vi "Router - PXImc Close.vi"(8 "error in (no error)":errorcluster, 11 "Router Data In":T1) -> (0 "error out":errorcluster)   [LabVIEW 2016, in "PXImc Router.lvlib"]
uses:
  PXImc Router.lvlib
  Controls/Router - Configuration.ctl
  Controls/Router/Node Block R-W Properties.ctl
  Controls/Router/Block Properties.ctl
  Controls/Router/Router - PXImc Properties.ctl
  Controls/Router/Router - PXImc Card Properties.ctl
  <vilib>/pximc/nipximc.lvlib
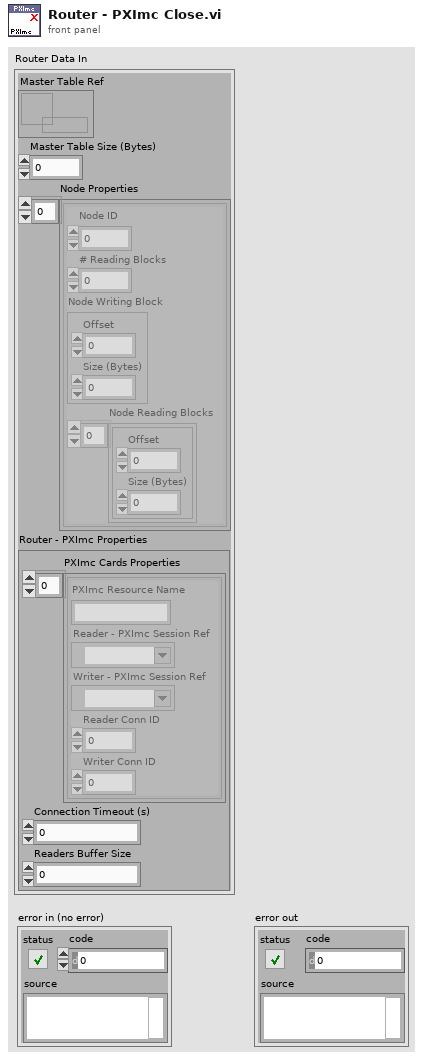
[diagram p1: front panel]
types:
  T1 = typedef "PXImc Router.lvlib/Router - Configuration.ctl" = cluster{"Master Table Ref":refnum<data-value>, "Master Table Size (Bytes)":u32, "Node Properties":T2[], "Router - PXImc Properties":T4}
  T2 = typedef "PXImc Router.lvlib/Node Block R-W Properties.ctl" = cluster{"Node ID":u32, "# Reading Blocks":u32, "Node Writing Block":T3, "Node Reading Blocks":T3[]}
  T3 = typedef "PXImc Router.lvlib/Block Properties.ctl" = cluster{"Offset":u32, "Size (Bytes)":u32}
  T4 = typedef "PXImc Router.lvlib/Router - PXImc Properties.ctl" = cluster{"PXImc Cards Properties":T5[], "Connection Timeout (s)":dbl, "Readers Buffer Size":u64}
  T5 = typedef "PXImc Router.lvlib/Router - PXImc Card Properties.ctl" = cluster{"PXImc Resource Name":string, "Reader - PXImc Session Ref":refnum<k21>, "Writer - PXImc Session Ref":refnum<k21>, "Reader Conn ID":u16, "Writer Conn ID":u16}
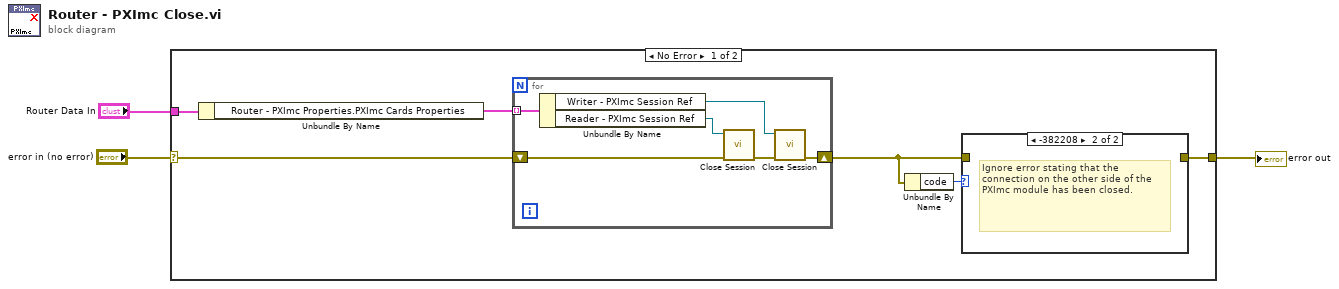
[diagram p0: block diagram]
diagram:
  n1 = case shown="No Error" "error in (no error)" {
    selector: "error in (no error)" -> [w6 w17]
    tunnel: [w7 w17] -> w2
    tunnel: "Router Data In" -> [w5 _]
    frame No Error {
      n2 = Unbundle By Name(w5) -> ("Router - PXImc Properties.PXImc Cards Properties"=w4:T5[])
      n3 = for {
        shift-right: [w15] -> w9
        shift-left: w6 -> [w14]
        tunnel: w4 -> [w12] mode=indexing
        n4 = Unbundle By Name(w12) -> ("Writer - PXImc Session Ref"=w10:refnum<k21>, "Reader - PXImc Session Ref"=w11:refnum<k21>)
        n5 = call <vilib>:"Close Session.vi"("error in (no error)"=w14, "session in"=w11) -> ("error out"=w13:errorcluster)  [unwired: 9 in]
        n6 = call <vilib>:"Close Session.vi"("error in (no error)"=w13, "session in"=w10) -> ("error out"=w15:errorcluster)  [unwired: 9 in]
      }
      n7 = Unbundle By Name(w9) -> ("code"=w8:i32)
      n8 = case shown="-382208" w8 {
        tunnel: w9 -> [w16 _]
        tunnel: [w16 _] -> w7
        frame 0, Default {
        }
        frame -382208 {
          # "Ignore error stating that the connection on the other side of the PXImc module has been closed."
        }
      }
    }
    frame Error {
    }
  }
  "error out" <- w2
